vi "cw_1_10.vi"() -> ()   [LabVIEW 2022 SP3]
panel:
  out "delta":dbl
  out "X2":cdb
  out "X1":cdb
  in  "C":dbl
  in  "B":dbl
  in  "A":dbl
  # "y(x) = Ax^2+Bx+C"
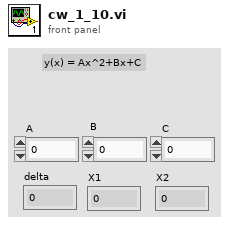
[diagram p1: front panel]
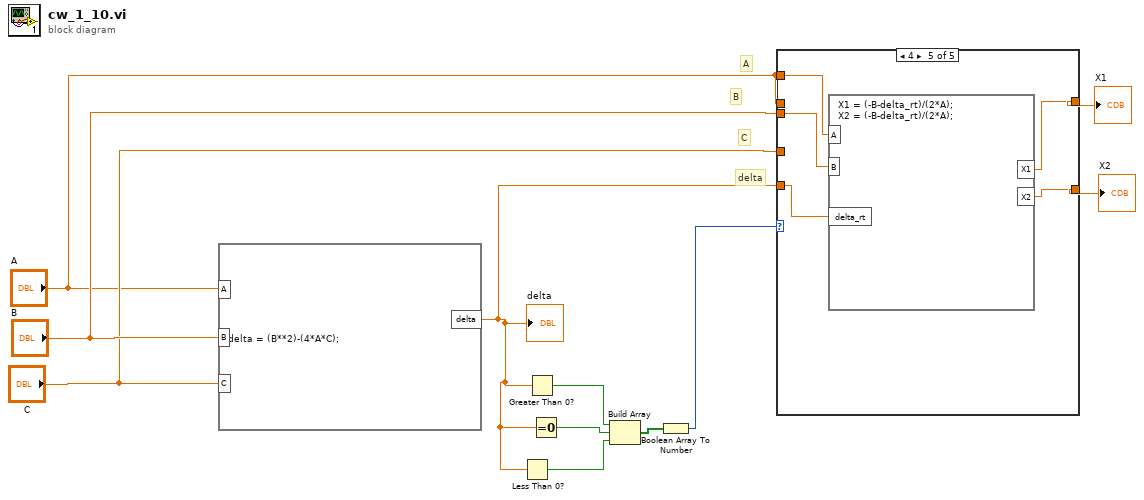
[diagram p0: block diagram]
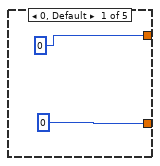
[diagram p2: hidden frame]
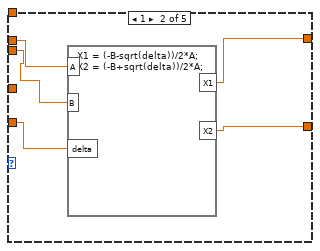
[diagram p3: hidden frame]
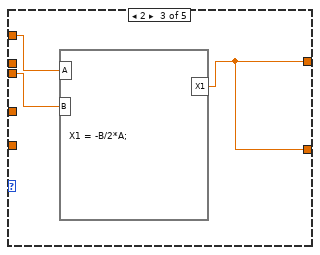
[diagram p4: hidden frame]
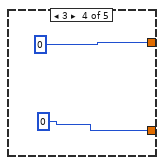
[diagram p5: hidden frame]
diagram:
  # "delta"
  # "C"
  # "B"
  # "A"
  n1 = formula code="delta = (B**2)-(4*A*C);"("C"="C", "B"="B", "A"="A") -> ("delta"=w5:dbl)
  "delta" <- w5
  n2 = Less Than 0?(x=w5) -> (x < 0?=w9:bool)
  n3 = Greater Than 0?(x=w5) -> (x > 0?=w11:bool)
  n4 = Equal To 0?(x=w5) -> (x = 0?=w10:bool)
  n5 = Build Array(w11, w10, w9) -> (w8:bool[])
  n6 = Boolean Array To Number(Boolean array=w8) -> (number=w1:u32)
  n7 = case shown="4" w1 {
    tunnel: "A" -> [_ _ w21 _ w26]
    tunnel: "B" -> [_ w17 w20 _ w27]
    tunnel: "C" -> [_ _ _ _ _]
    tunnel: w5 -> [_ w16 _ _ w28]
    tunnel: [0 w15 w19 0 w24] -> w4
    tunnel: [0 w14 w19 0 w25] -> w3
    tunnel: "A" -> [_ w18 _ _ _]
    frame 0, Default {
    }
    frame 1 {
      n8 = formula code="X1 = (-B-sqrt(delta))/2*A;\nX2 = (-B+sqrt(delta))/2*A;"("A"=w18, "B"=w17, "delta"=w16) -> ("X1"=w15:dbl, "X2"=w14:dbl)
    }
    frame 2 {
      n9 = formula code="X1 = -B/2*A;"("A"=w21, "B"=w20) -> ("X1"=w19:dbl)
    }
    frame 3 {
    }
    frame 4 {
      n10 = formula code="X1 = (-B-delta_rt)/(2*A);\nX2 = (-B-delta_rt)/(2*A);"("A"=w26, "B"=w27, "delta_rt"=w28) -> ("X1"=w24:dbl, "X2"=w25:dbl)
    }
  }
  "X1" <- w4
  "X2" <- w3
